vi "build_error_cluster.vi"(8 "error in (no error)":errorcluster, 9 "error msg (JSON)":string, 10 "status code":string, 11 "headers array":string[](array[string])) -> (0 "error out":errorcluster)   [LabVIEW 2018]
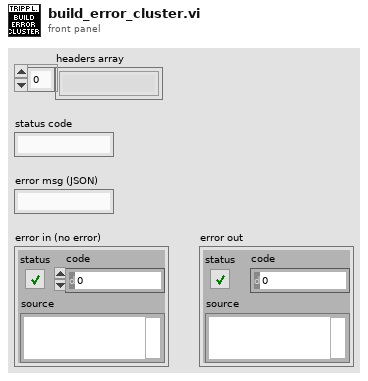
[diagram p1: front panel]
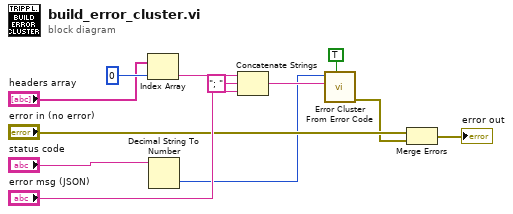
[diagram p0: block diagram]
diagram:
  n1 = Index Array(array="headers array", index=0) -> (element=w9:string)
  n2 = Decimal String To Number(string="status code") -> (number=w2:i32)  [unwired: 2 in, 1 out]
  n3 = Concatenate Strings(w9, "; " ("string"), "error msg (JSON)") -> (w12:string)
  n4 = call <vilib>:"Error Cluster From Error Code.vi"("show call chain? (False)"=TRUE, "error message (\"\")"=w12, "error code (0)"=w2) -> ("error out"=w6:errorcluster)  [unwired: 6 in]
  n5 = Merge Errors("error in (no error)", w6) -> (→"error out":errorcluster)
